vi "例程17-设计一个颜色表.vi"() -> ()   [LabVIEW 2016]
panel:
  out "添加的数组":u32[](array[numeric])
  in  "停止":bool
  in  "下溢颜色":u32(colorbox)
  in  "上溢颜色":u32(colorbox)
  in  "颜色表":u32(colorbox)
  out "强度图":i32[][](graph)
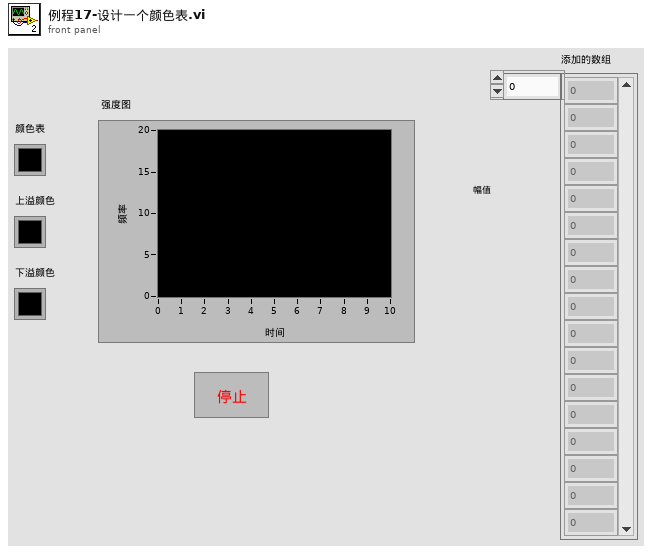
[diagram p1: front panel]
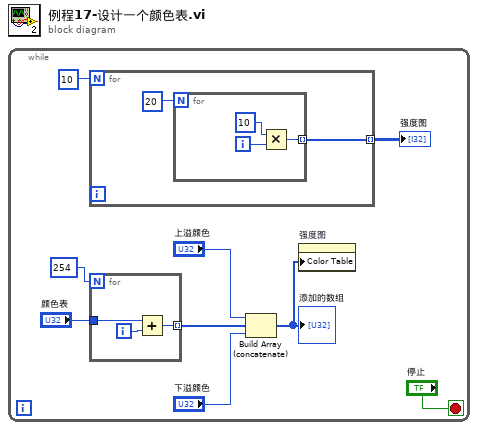
[diagram p0: block diagram]
diagram:
  n1 = while {
    stop <- "停止" stop-if-true
    n2 = for {
      N: 10 -> [_]
      tunnel: [w11] -> w9 mode=indexing
      n3 = for {
        N: 20 -> [_]
        tunnel: [w12] -> w11 mode=indexing
        i -> [w14]
        n4 = Multiply(x=10, y=w14) -> (x*y=w12:i32)
      }
    }
    "强度图" <- w9
    n5 = for {
      N: 254 -> [_]
      tunnel: "颜色表" -> [w16]
      tunnel: [w15] -> w7 mode=indexing
      i -> [w17]
      n6 = Add(x=w16, y=w17) -> (x+y=w15:u32)
    }
    n7 = Build Array (concatenate)("上溢颜色", w7, "下溢颜色") -> (w2:u32[])
    "添加的数组" <- w2
    n8 = property on="强度图" class="IntGraph (严格)"("Color Table"=w2) -> ()  [unwired: 2 in, 2 out]
  }
